vi "Detect Correlation.vi"(10 "frequency":dbl, 11 "Signal":dbl[](array[numeric])) -> (3 "Output":dbl)   [LabVIEW 2014]
uses:
  <vilib>/measure/NI_MAPro.lvlib
panel:
  out "x*y":dbl[](array[numeric])
  out "sum":dbl
  out "error out 2":errorcluster
  out "error out":errorcluster
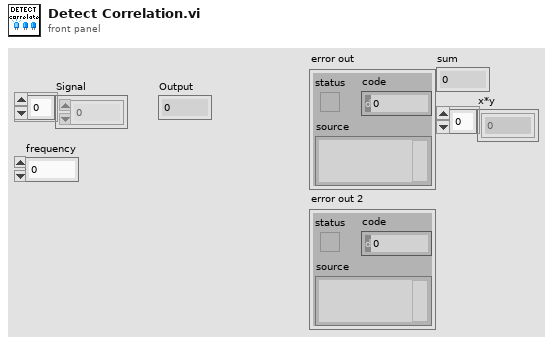
[diagram p1: front panel]
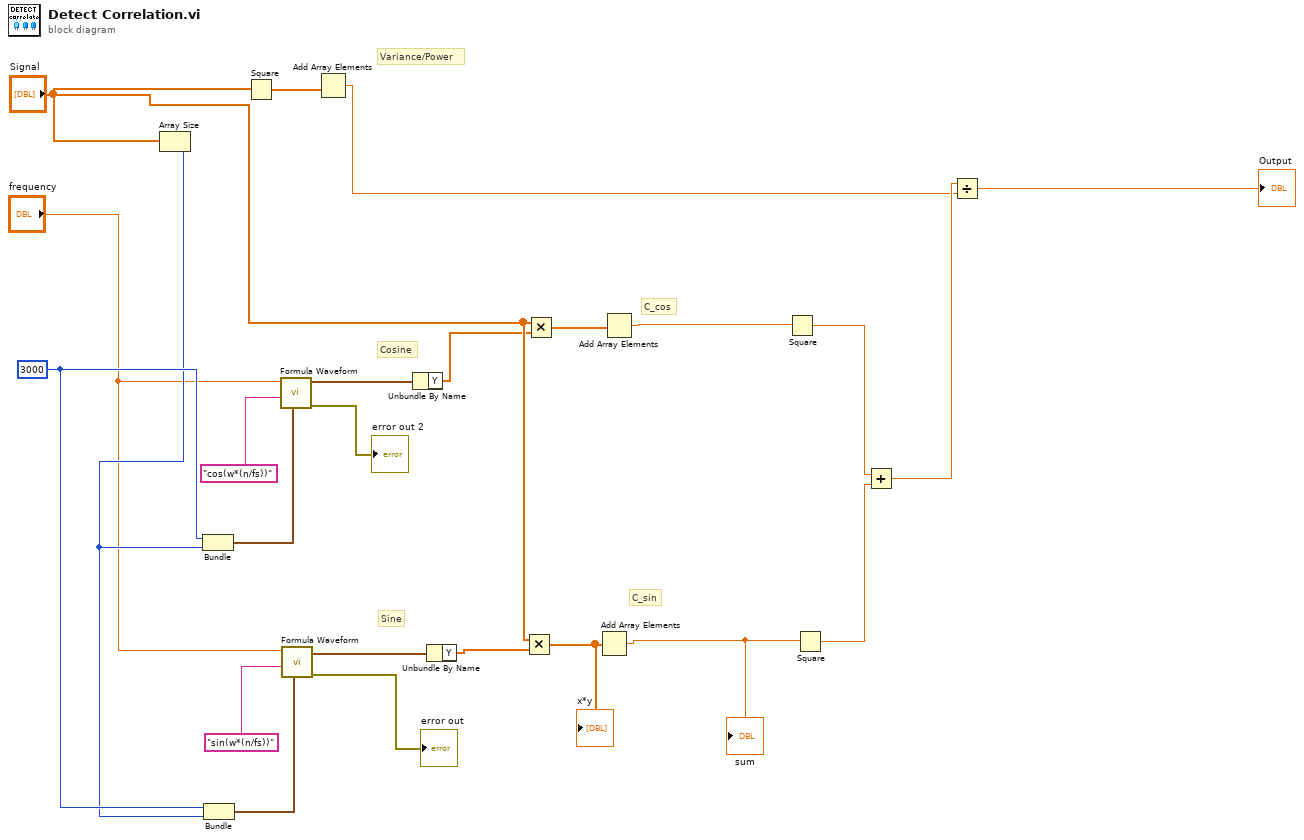
[diagram p0: block diagram]
diagram:
  w22 = 3000
  # "C_sin"
  # "C_cos"
  # "Variance/Power"
  # "Sine"
  # "Cosine"
  n1 = Array Size(array="Signal") -> (size(s)=w21:i32)
  n2 = Bundle(w22, w21) -> (w2:cluster{i32, i32})  [unwired: 1 in]
  n3 = Bundle(w22, w21) -> (w1:cluster{i32, i32})  [unwired: 1 in]
  n4 = Square(x="Signal") -> (x^2=w17:dbl[])
  n5 = call <vilib>:"Formula Waveform.vi"("sampling info"=w2, "formula"="cos(w*(n/fs))", "frequency"="frequency") -> ("error out"=→"error out 2":errorcluster, "signal out"=w18:waveform(dbl))  [unwired: 7 in]
  n6 = call <vilib>:"Formula Waveform.vi"("sampling info"=w1, "formula"="sin(w*(n/fs))", "frequency"="frequency") -> ("error out"=→"error out":errorcluster, "signal out"=w19:waveform(dbl))  [unwired: 7 in]
  n7 = Add Array Elements(numeric array=w17) -> (sum=w7:dbl)
  n8 = Unbundle By Name(w18) -> ("Y"=w5:dbl[])
  n9 = Unbundle By Name(w19) -> ("Y"=w16:dbl[])
  n10 = Multiply(x="Signal", y=w16) -> (x*y=w14:dbl[])
  "x*y" <- w14
  n11 = Multiply(x="Signal", y=w5) -> (x*y=w13:dbl[])
  n12 = Add Array Elements(numeric array=w14) -> (sum=w12:dbl)
  "sum" <- w12
  n13 = Add Array Elements(numeric array=w13) -> (sum=w10:dbl)
  n14 = Square(x=w10) -> (x^2=w9:dbl)
  n15 = Square(x=w12) -> (x^2=w11:dbl)
  n16 = Add(x=w9, y=w11) -> (x+y=w8:dbl)
  n17 = Divide(x=w8, y=w7) -> (x/y=→"Output":dbl)
